vi "GDSLvClass_GetLibraryItemFromPath.vi"(0 "Library Refnum In":refnum<vi>, 1 "VINames":path, 5 "error in (no error)":errorcluster) -> (14 "Item Refnum Out":refnum<vi>, 19 "error out":errorcluster)   [LabVIEW 2014]
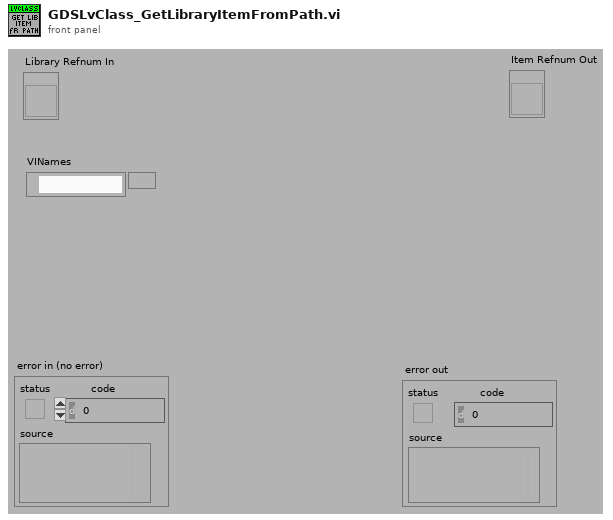
[diagram p1: front panel]
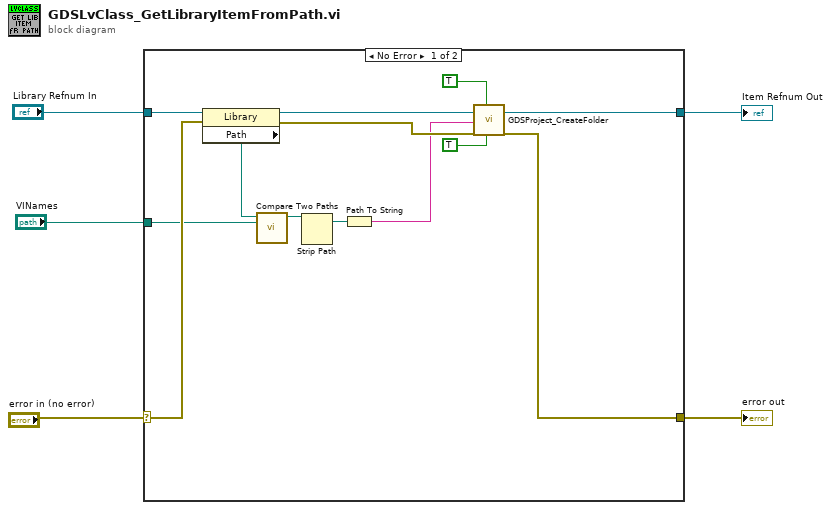
[diagram p0: block diagram]
diagram:
  n1 = case shown="No Error" "error in (no error)" {
    selector: "error in (no error)" -> [w17 w19]
    tunnel: [w6 w19] -> w4
    tunnel: "Library Refnum In" -> [w18 _]
    tunnel: [w7 _] -> w2
    tunnel: "VINames" -> [w15 _]
    frame No Error {
      n2 = property class="Library"(reference=w18, error in=w17) -> (reference out=w13:refnum<vi>, error out=w12:errorcluster, "Path"=w16:path)
      n3 = call <vilib>:"Compare Two Paths.vi"("Path 2"=w15, "Path 1"=w16) -> ("Relative Path from 1 to 2"=w14:path)  [unwired: 6 in, 3 out]
      n4 = Strip Path(path=w14) -> (stripped path=w11:path)  [unwired: 1 out]
      n5 = Path To String(path=w11) -> (string=w10:string)
      n6 = call <resource>:"GDSProject_CreateFolder.vi"("Project Item To Create Folder Below(Use MyComputer if not wired)"=w13, "FolderName"=w10, "error in (no error)"=w12, "CreateThePhysicalFolderIfPossible(False)"=TRUE, "GuessFolderScope(False)"=TRUE) -> ("ItemOut"=w7:refnum<vi>, "error out"=w6:errorcluster)  [unwired: 11 in, 2 out]
    }
    frame Error {
    }
  }
  "Item Refnum Out" <- w2
  "error out" <- w4
